vi "Pull from Stream.vi"(8 "error in (no error)":errorcluster, 11 "stream in":refnum<queue>) -> (0 "error out":errorcluster, 2 "element":T1, 3 "queue out":refnum<queue>)   [LabVIEW 2014]
uses:
  Action/Action.ctl
  Action/Action Name.ctl
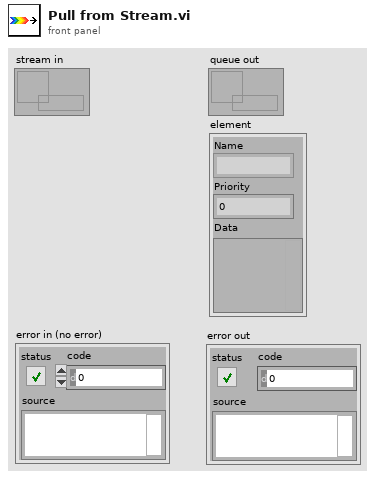
[diagram p1: front panel]
types:
  T1 = typedef "Action.ctl" = cluster{"Name":T2, "Priority":i32, "Data":variant}
  T2 = typedef "Action Name.ctl" = enum16{""}
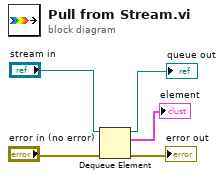
[diagram p0: block diagram]
diagram:
  n1 = Dequeue Element(queue="stream in", error in (no error)="error in (no error)") -> (queue out=→"queue out":refnum<queue>, element=→"element":T1, error out=→"error out":errorcluster)  [unwired: 1 in, 1 out]
